vi "Sum Mass Element Matrix for Accelerometer.vi"(9 "Matrix w/o BC":dbl[][](array[numeric]), 10 "accelerometer_mass":dbl, 11 "Element Length":dbl) -> (3 "Matrix W/ Accelerometer":dbl[][](array[numeric]))   [LabVIEW 2021]
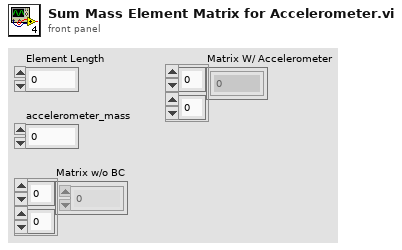
[diagram p1: front panel]
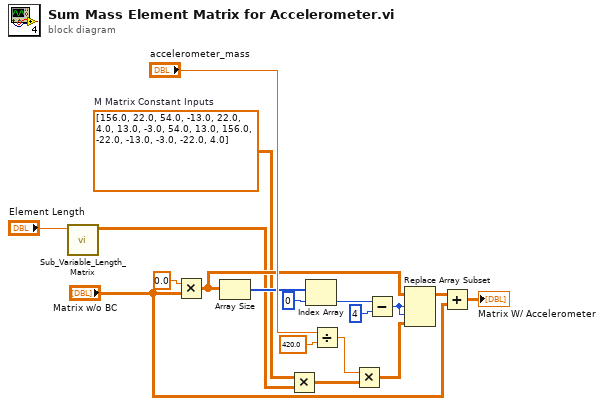
[diagram p0: block diagram]
diagram:
  w6 = dbl[][] [[156.0, 22.0, 54.0, -13.0], [22.0, 4.0, 13.0, -3.0], [54.0, 13.0, 156.0, -22.0], [-13.0, -3.0, -22.0, 4.0]]  # M Matrix Constant Inputs
  n1 = call "Sub_Variable_Length_Matrix.vi"("Numeric"="Element Length") -> ("Array"=w8:dbl[][])  [unwired: 10 in]
  n2 = Multiply(x=0.0, y="Matrix w/o BC") -> (x*y=w10:dbl[][])
  n3 = Array Size(array=w10) -> (size(s)=w11:i32[])
  n4 = Multiply(x=w6, y=w8) -> (x*y=w5:dbl[][])
  n5 = Index Array(array=w11, index=0) -> (element=w13:i32)
  n6 = Divide(x="accelerometer_mass", y=420.0) -> (x/y=w4:dbl)
  n7 = Multiply(x=w4, y=w5) -> (x*y=w16:dbl[][])
  n8 = Subtract(x=w13, y=4) -> (x-y=w15:i32)
  n9 = Replace Array Subset(array=w10, new element=w16, index (row)=w15, index (col)=w15) -> (w17:dbl[][])
  n10 = Add(x=w17, y="Matrix w/o BC") -> (x+y=→"Matrix W/ Accelerometer":dbl[][])
